vi "thorlabs_move_piezos.vi"(8 "error in (no error)":errorcluster, 10 "new_positions":dbl[](array[numeric]), 11 "thorlabs_panel in":refnum<class "thorlabs_panel.lvclass">) -> (0 "error out":errorcluster, 3 "thorlabs_panel out":refnum<class "thorlabs_panel.lvclass">)   [LabVIEW 2015, in "thorlabs_panel.lvclass"]
uses:
  thorlabs_panel.lvclass
  thorlabs_class/thorlabs_kinesis.lvclass
  UI/panel_class/panel.lvclass
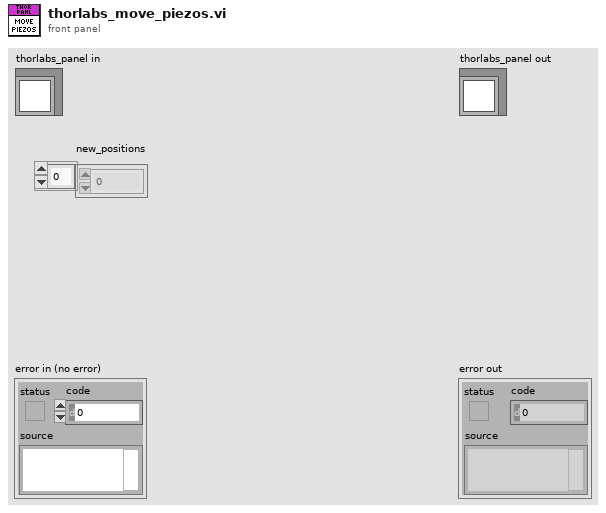
[diagram p1: front panel]
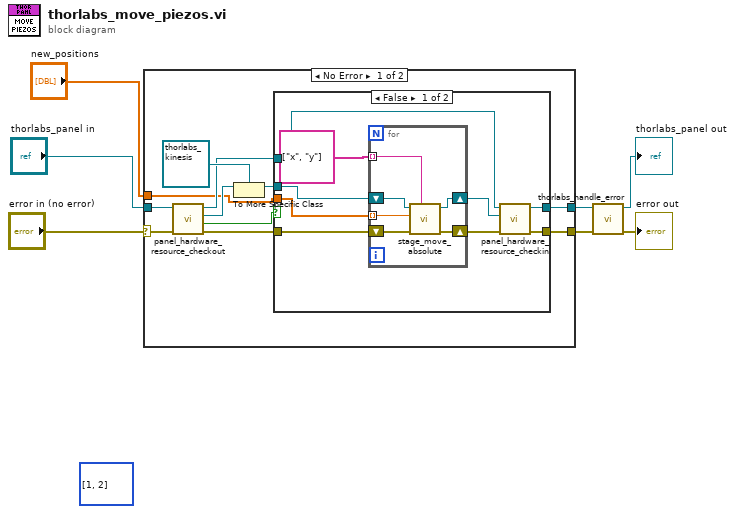
[diagram p0: block diagram]
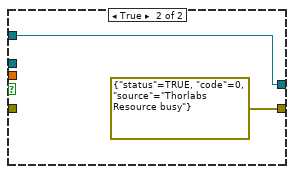
[diagram p2: hidden frame]
diagram:
  (unwired) i32[] [1, 2]
  n1 = case shown="No Error" "error in (no error)" {
    selector: "error in (no error)" -> [w17 w37]
    tunnel: [w9 w37] -> w1
    tunnel: [w8 w36] -> w4
    tunnel: "thorlabs_panel in" -> [w18 w36]
    tunnel: "new_positions" -> [w10 _]
    frame No Error {
      n2 = call "panel_hardware_resource_checkout.vi"("error in (no error)"=w17, "panel in"=w18) -> ("error out"=w13:errorcluster, "timed out?"=w12:bool, "hardware.lvclass"=w16:refnum<class "hardware.lvclass">, "panel out"=w11:refnum<class "thorlabs_panel.lvclass">)  [unwired: 6 in]
      n3 = To More Specific Class(target class=refnum<class "thorlabs_kinesis.lvclass"> refnum ("thorlabs_kinesis.lvclass"), reference=w16) -> (specific class reference=w14:refnum<class "thorlabs_kinesis.lvclass">)  [unwired: 1 in, 1 out]
      n4 = case shown="False" w12 {
        tunnel: w14 -> [w22 _]
        tunnel: w13 -> [w23 _]
        tunnel: w11 -> [w25 w34]
        tunnel: [w27 w34] -> w8
        tunnel: [w26 errorcluster {"status"=TRUE, "code"=0, "source"="Thorlabs Resource busy"} ("error out")] -> w9
        tunnel: w10 -> [w24 _]
        frame False {
          n5 = for {
            tunnel: string[] ["x", "y"] -> [w33] mode=indexing
            tunnel: w24 -> [w32] mode=indexing
            shift-right: [w29] -> w21
            shift-left: w23 -> [w31]
            shift-right: [w28] -> w20
            shift-left: w22 -> [w30]
            n6 = call-dynamic "stage_move_absolute.vi"("Stage Name"=w33, "error in (no error)"=w31, "Position"=w32, "Stage in"=w30) -> ("error out"=w29:errorcluster, "Stage out"=w28:refnum<class "thorlabs_kinesis.lvclass">)  [unwired: 6 in]
          }
          n7 = call "panel_hardware_resource_checkin.vi"("error in (no error)"=w21, "hardware.lvclass"=w20, "panel in"=w25) -> ("error out"=w26:errorcluster, "panel out"=w27:refnum<class "thorlabs_panel.lvclass">)  [unwired: 7 in]
        }
        frame True {
        }
      }
    }
    frame Error {
    }
  }
  n8 = call "thorlabs_handle_error.vi"("error in (no error)"=w1, "thorlabs_panel in"=w4) -> ("error out"=→"error out":errorcluster, "thorlabs_panel out"=→"thorlabs_panel out":refnum<class "thorlabs_panel.lvclass">)  [unwired: 8 in]
